vi "Get Extension.vi"(2 "Path In":path) -> (7 "Duplicate Path Out":path, 9 "Extension":string)   [LabVIEW 2012, in "paint Xcontrol.xctl"]
uses:
  paint Xcontrol.xctl
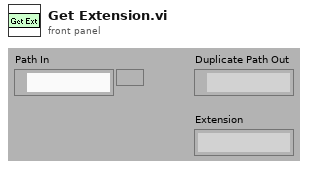
[diagram p1: front panel]
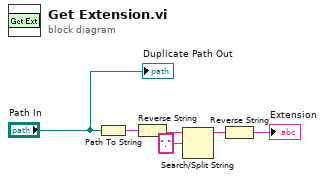
[diagram p0: block diagram]
diagram:
  n1 = Path To String(path="Path In") -> (string=w2:string)
  n2 = Reverse String(1:w2) -> (0:w3:string)
  n3 = Search/Split String(string=w3, search string/char (-)=".") -> (substring before match=w5:string)  [unwired: 1 in, 2 out]
  n4 = Reverse String(1:w5) -> (0:→"Extension":string)
  "Duplicate Path Out" <- "Path In"
